vi "Variant Array Reshape.vi"(8 "error in (no error)":errorcluster, 9 "Default Element Type":variant, 10 "Sizes":i32[](array[numeric]), 11 "Elements":variant[](array[variant])) -> (0 "error out":errorcluster, 3 "N Dim Array":variant)   [LabVIEW 2018, in "labview_json.lvlib"]
uses:
  labview_json.lvlib
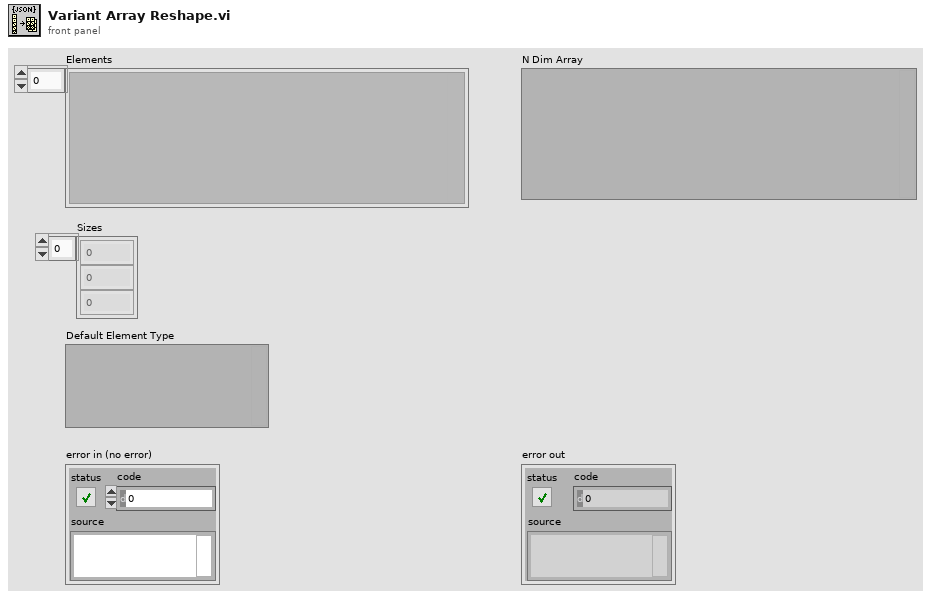
[diagram p1: front panel]
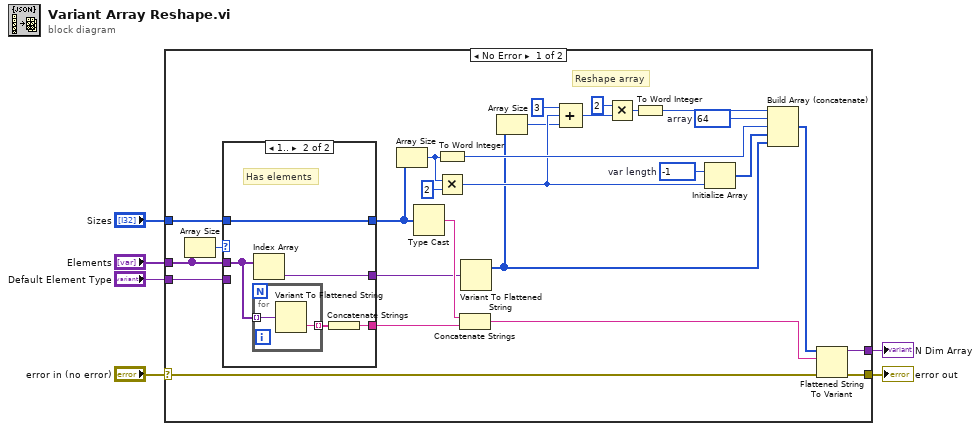
[diagram p0: block diagram]
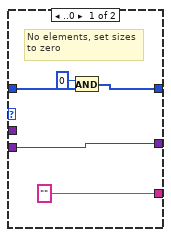
[diagram p2: hidden frame]
diagram:
  n1 = case shown="No Error" "error in (no error)" {
    selector: "error in (no error)" -> [w14 w46]
    tunnel: [w33 w46] -> w5
    tunnel: "Elements" -> [w12 _]
    tunnel: [w32 _] -> w3
    tunnel: "Sizes" -> [w7 _]
    tunnel: "Default Element Type" -> [w9 _]
    frame No Error {
      w23 = i16 -1  # var length
      w29 = i16 64  # array
      # "Reshape array"
      n2 = Array Size(array=w12) -> (size(s)=w13:i32)
      n3 = case shown="1.." w13 {
        tunnel: w12 -> [_ w43]
        tunnel: ["" w40] -> w10
        tunnel: [w38 w41] -> w11
        tunnel: w9 -> [w38 _]
        tunnel: [w35 w39] -> w8
        tunnel: w7 -> [w34 w39]
        frame ..0 {
          # "No elements, set sizes\nto zero"
          n4 = And(x=0, y=w34) -> (x .and. y?=w35:i32[])
        }
        frame 1.. {
          # "Has elements"
          n5 = for {
            tunnel: w43 -> [w45] mode=indexing
            tunnel: [w44] -> w42 mode=indexing
            n6 = Variant To Flattened String(Variant=w45) -> (data string=w44:string)  [unwired: 1 out]
          }
          n7 = Index Array(array=w43) -> (element=w41:variant)  [unwired: 1 in]
          n8 = Concatenate Strings(w42) -> (w40:string)
        }
      }
      n9 = Array Size(array=w8) -> (size(s)=w25:i32)
      n10 = Type Cast(x=w8) -> (*(type *) &x=w27:string)  [unwired: 1 in]
      n11 = To Word Integer(number=w25) -> (16bit integer=w24:i16)
      n12 = Multiply(x=w25, y=2 ("x")) -> (x*y=w22:i32)
      n13 = Concatenate Strings(w27, w10) -> (w26:string)
      n14 = Variant To Flattened String(Variant=w11) -> (1:w15:i16[])  [unwired: 1 out]
      n15 = Array Size(array=w15) -> (size(s)=w16:i32)
      n16 = Compound Arithmetic op=ADD(3 ("x"), w22, w16) -> (w19:i32)
      n17 = Multiply(x=2, y=w19) -> (x*y=w18:i32)
      n18 = To Word Integer(number=w18) -> (16bit integer=w17:i16)
      n19 = Initialize Array(w23, w22) -> (w21:i16[])
      n20 = Build Array (concatenate)(w17, w29, w24, w21, w15) -> (w28:i16[])
      n21 = Flattened String To Variant(4:w14, 6:w26, 7:w28) -> (0:w33:errorcluster, 3:w32:variant)
    }
    frame Error {
    }
  }
  "error out" <- w5
  "N Dim Array" <- w3
